vi "Set Device Name.vi"(8 "error in (no error)":errorcluster, 10 "Name":string, 11 "EPU452 in":refnum<class "EPU452.lvclass">) -> (0 "error out":errorcluster, 2 "Response":string, 3 "EPU452 out":refnum<class "EPU452.lvclass">)   [LabVIEW 2018, in "EPU452.lvclass"]
uses:
  EPU452.lvclass
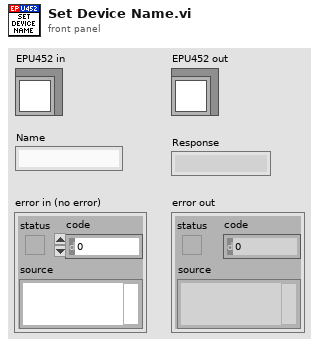
[diagram p1: front panel]
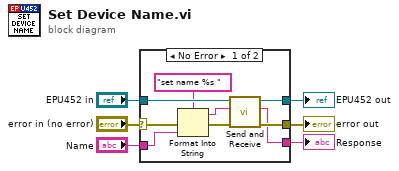
[diagram p0: block diagram]
diagram:
  n1 = case shown="No Error" "error in (no error)" {
    selector: "error in (no error)" -> [w11 w17]
    tunnel: [w13 w17] -> w5
    tunnel: [w14 w16] -> w3
    tunnel: "EPU452 in" -> [w15 w16]
    tunnel: "Name" -> [w8 _]
    tunnel: [w7 _] -> w1
    frame No Error {
      n2 = Format Into String(format string="set name %s " ("string"), error in=w11, w8) -> (resulting string=w10:string, error out=w12:errorcluster)  [unwired: 1 in]
      n3 = call "Send and Receive.vi"("error in (no error)"=w12, "Command"=w10, "EPU452 in"=w15) -> ("error out"=w13:errorcluster, "Response"=w7:string, "EPU452 out"=w14:refnum<class "EPU452.lvclass">)  [unwired: 6 in]
    }
    frame Error {
    }
  }
  "error out" <- w5
  "EPU452 out" <- w3
  "Response" <- w1
